vi "Configure Modulation (FM).vi"(0 "VISA resource name":refnum<visa-resource-name>, 1 "Enable Frequency Modulation (T:Enable)":bool=TRUE, 2 "Modulation Waveform (0: Sine)":u16(ring) items=["Sine", "Square", "Triangle", "UpRamp", "DnRamp", "Noise", "Arb"], 5 "FM Source (0: Internal)":u16(ring) items=["Internal", "External"], 7 "Channel (1:Channel 1)":i32(ring)=1 items=["Channel 1"=1, "Channel 2"=2], 9 "FM Deviation (100.000 Hz)":dbl=100.0 format="%.3f", 11 "error in (no error)":errorcluster, 12 "Modulation Frequency (100.000 Hz)":dbl=100.0 format="%.3f") -> (4 "VISA resource name out":refnum<visa-resource-name>, 15 "error out":errorcluster)   [LabVIEW 2022 SP3, in "Siglent SDG X Series.lvlib"]
doc: "Configures and enables frequency modulation (FM). In FM, the frequency of the carrier is varied by the frequency of the modulating waveform. \n\n<B>Note:</B> The carrier waveform shape and parameters are set by the Configure Standard Waveform VI."
uses:
  Siglent SDG X Series.lvlib
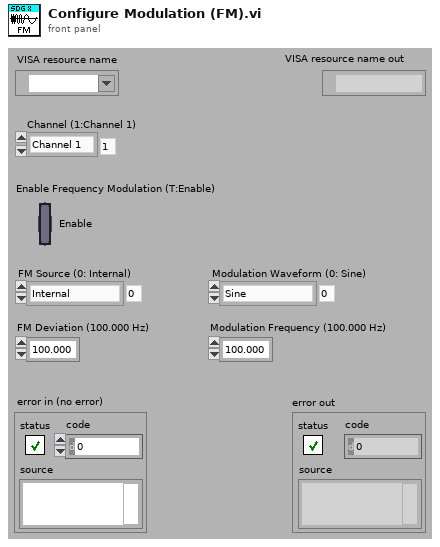
[diagram p1: front panel]
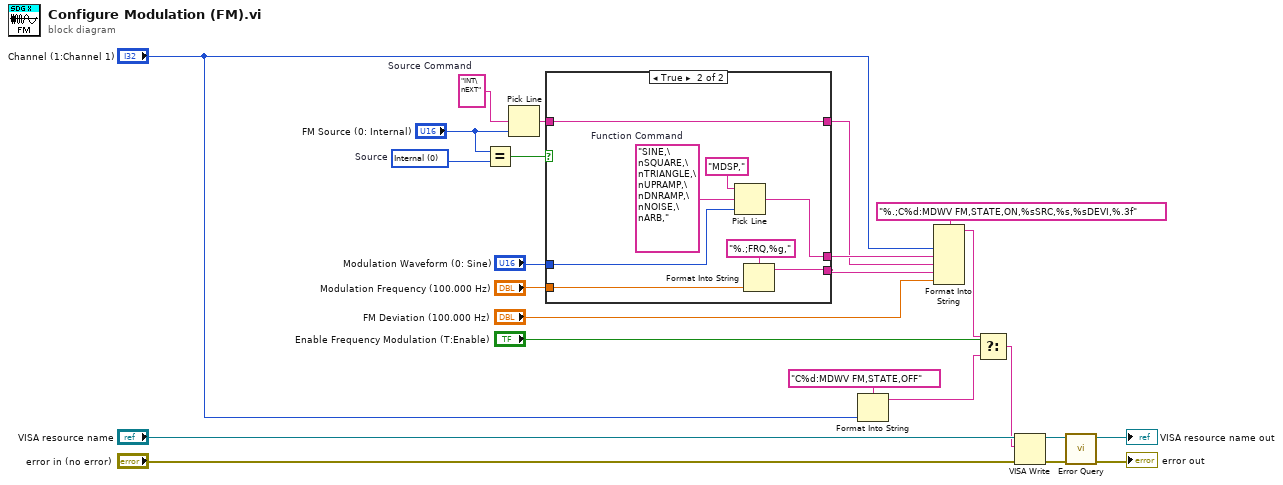
[diagram p0: block diagram]
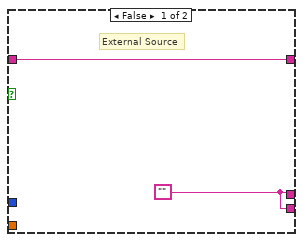
[diagram p2: hidden frame]
diagram:
  w17 = "INT\nEXT"  # Source Command
  w8 = u16 0 items=["Internal", "External"]  # Source
  n1 = Equal?(x="FM Source (0: Internal)", y=w8) -> (x = y?=w16:bool)
  n2 = Pick Line(multi-line string=w17, line index="FM Source (0: Internal)") -> (output string=w15:string)  [unwired: 1 in]
  n3 = case shown="True" w16 {
    tunnel: w15 -> [w26 w32]
    tunnel: "Modulation Waveform (0: Sine)" -> [_ w33]
    tunnel: "Modulation Frequency (100.000 Hz)" -> [_ w29]
    tunnel: [w26 w32] -> w12
    tunnel: [w25 w30] -> w13
    tunnel: [w25 w27] -> w11
    frame False {
      w25 = ""
      # "External Source"
    }
    frame True {
      w34 = "SINE,\nSQUARE,\nTRIANGLE,\nUPRAMP,\nDNRAMP,\nNOISE,\nARB,"  # Function Command
      n4 = Pick Line(string ("")="MDSP,", multi-line string=w34, line index=w33) -> (output string=w30:string)
      n5 = Format Into String(format string="%.;FRQ,%g,", w29) -> (resulting string=w27:string)  [unwired: 2 in, 1 out]
    }
  }
  n6 = Format Into String(format string="C%d:MDWV FM,STATE,OFF", "Channel (1:Channel 1)") -> (resulting string=w3:string)  [unwired: 2 in, 1 out]
  n7 = Format Into String(format string="%.;C%d:MDWV FM,STATE,ON,%sSRC,%s,%sDEVI,%.3f", "Channel (1:Channel 1)", w13, w12, w11, "FM Deviation (100.000 Hz)") -> (resulting string=w4:string)  [unwired: 2 in, 1 out]
  n8 = Select(t=w4, s="Enable Frequency Modulation (T:Enable)", f=w3) -> (s? t:f=w2:string)
  n9 = VISA Write(VISA resource name="VISA resource name", write buffer=w2, error in (no error)="error in (no error)") -> (VISA resource name out=w22:refnum<visa-resource-name>, error out=w21:errorcluster)  [unwired: 1 out]
  n10 = call "Error Query.vi"("error in (no error)"=w21, "VISA resource name"=w22) -> ("error out"=→"error out":errorcluster, "VISA resource name out"=→"VISA resource name out":refnum<visa-resource-name>)  [unwired: 6 in, 2 out]
